vi "CalcVectors.vi"(8 "In/out":dbl, 9 "Up/down":dbl, 10 "Shoulder Degrees":dbl, 11 "Elbow Degrees":dbl) -> (2 "Shoulder Power":dbl, 3 "Elbow power":dbl)   [LabVIEW 2018]
panel:
  out "Theta C 2":dbl
  out "Theta b 2":dbl
  out "sin(b) 2":dbl
  out "sin(c) 2":dbl
  out "sin(b)":dbl
  out "sin(c)":dbl
  out "Theta C":dbl
  out "Theta b":dbl
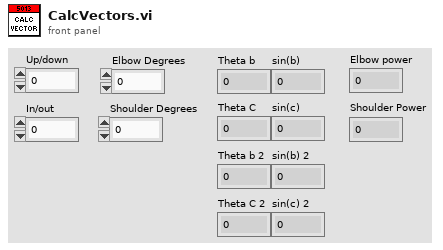
[diagram p1: front panel]
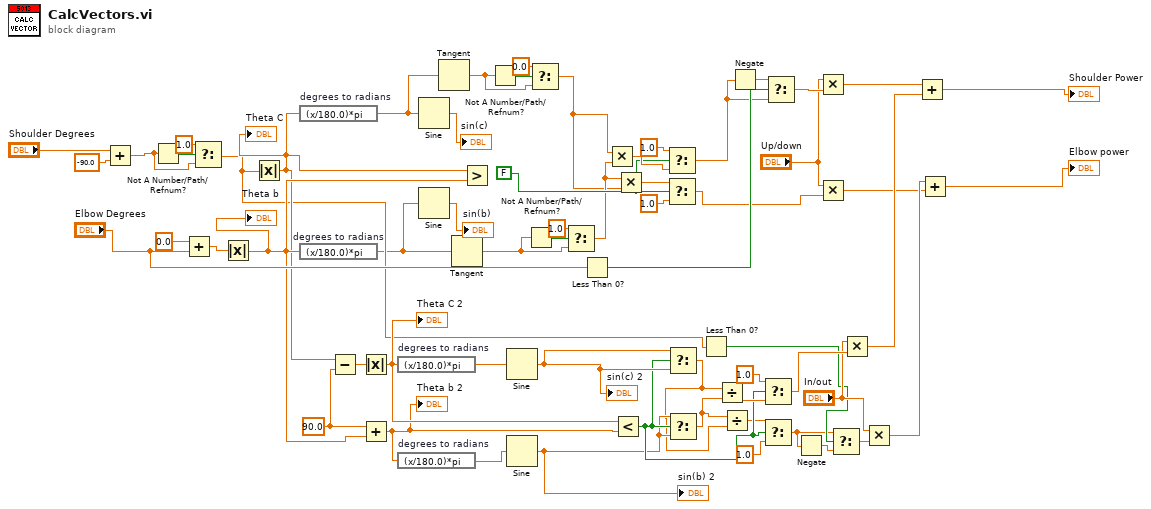
[diagram p0: block diagram]
diagram:
  w13 = FALSE
  w45 = 90.0 ("x")
  n1 = Add(x="Shoulder Degrees", y=-90.0) -> (x+y=w15:dbl)
  n2 = Not A Number/Path/Refnum?(number/path/refnum=w15) -> (NaN/Path/Refnum?=w17:bool)
  n3 = Add(x=0.0, y="Elbow Degrees") -> (x+y=w39:dbl)
  n4 = Select(t=1.0, s=w17, f=w15) -> (s? t:f=w16:dbl)
  n5 = Absolute Value(x=w39) -> (abs(x)=w19:dbl)
  "Theta b" <- w19
  n6 = Absolute Value(x=w16) -> (abs(x)=w18:dbl)
  "Theta C" <- w18
  n7 = expression code="(x/180.0)*pi" "degrees to radians"(w18) -> (w10:dbl)
  n8 = expression code="(x/180.0)*pi" "degrees to radians"(w19) -> (w12:dbl)
  n9 = Subtract(x=w18, y=w45) -> (x-y=w44:dbl)
  n10 = Absolute Value(x=w44) -> (abs(x)=w37:dbl)
  "Theta C 2" <- w37
  n11 = Add(x=w45, y=w19) -> (x+y=w36:dbl)
  "Theta b 2" <- w36
  n12 = expression code="(x/180.0)*pi" "degrees to radians"(w37) -> (w52:dbl)
  n13 = expression code="(x/180.0)*pi" "degrees to radians"(w36) -> (w51:dbl)
  n14 = Sine(x=w10) -> (sin(x)=→"sin(c)":dbl)
  n15 = Sine(x=w12) -> (sin(x)=→"sin(b)":dbl)
  n16 = Tangent(1:w10) -> (0:w2:dbl)
  n17 = Tangent(1:w12) -> (0:w5:dbl)
  n18 = Greater?(x=w18, y=w19) -> ()  [unwired: 1 out]
  n19 = Not A Number/Path/Refnum?(number/path/refnum=w2) -> (NaN/Path/Refnum?=w4:bool)
  n20 = Sine(x=w52) -> (sin(x)=w50:dbl)
  "sin(c) 2" <- w50
  n21 = Sine(x=w51) -> (sin(x)=w40:dbl)
  "sin(b) 2" <- w40
  n22 = Not A Number/Path/Refnum?(number/path/refnum=w5) -> (NaN/Path/Refnum?=w7:bool)
  n23 = Select(t=0.0, s=w4, f=w2) -> (s? t:f=w1:dbl)
  n24 = Select(t=1.0, s=w7, f=w5) -> (s? t:f=w6:dbl)
  n25 = Less Than 0?(x="Elbow Degrees") -> (x < 0?=w35:bool)
  n26 = Multiply(x=w1, y=w6) -> (x*y=w20:dbl)
  n27 = Less?(x=w37, y=w36) -> (x < y?=w43:bool)
  n28 = Multiply(x=w6, y=w1) -> (x*y=w21:dbl)
  n29 = Select(t=1.0, s=w13, f=w20) -> (s? t:f=w29:dbl)
  n30 = Select(t=w21, s=w13, f=1.0) -> (s? t:f=w28:dbl)
  n31 = Select(t=w50, s=w43, f=w50) -> (s? t:f=w32:dbl)
  n32 = Select(t=w40, s=w43, f=w40) -> (s? t:f=w33:dbl)
  n33 = Less Than 0?(x=w16) -> (x < 0?=w26:bool)
  n34 = Divide(x=w32, y=w33) -> (x/y=w49:dbl)
  n35 = Divide(x=w33, y=w32) -> (x/y=w34:dbl)
  n36 = Negate(x=w29) -> (-x=w22:dbl)
  n37 = Select(t=1.0, s=w43, f=w49) -> (s? t:f=w47:dbl)
  n38 = Select(t=w34, s=w43, f=1.0) -> (s? t:f=w25:dbl)
  n39 = Select(t=w22, s=w35, f=w29) -> (s? t:f=w54:dbl)
  n40 = Negate(x=w25) -> (-x=w24:dbl)
  n41 = Multiply(x="Up/down", y=w54) -> (x*y=w30:dbl)
  n42 = Multiply(x="Up/down", y=w28) -> (x*y=w31:dbl)
  n43 = Select(t=w25, s=w26, f=w24) -> (s? t:f=w27:dbl)
  n44 = Multiply(x="In/out", y=w47) -> (x*y=w41:dbl)
  n45 = Multiply(x="In/out", y=w27) -> (x*y=w57:dbl)
  n46 = Add(x=w30, y=w41) -> (x+y=→"Shoulder Power":dbl)
  n47 = Add(x=w57, y=w31) -> (x+y=→"Elbow power":dbl)
